vi "Add Library To Project.vi"(8 "error in":errorcluster, 11 "Msg Script Strategy in":refnum<class "Msg Script Strategy.lvclass">) -> (0 "error out":errorcluster)   [LabVIEW 2021, in "_Create From Template.lvlib" / "Script Strategy.lvlib" / "Msg Script Strategy.lvclass"]
uses:
  Msg Script Strategy.lvclass
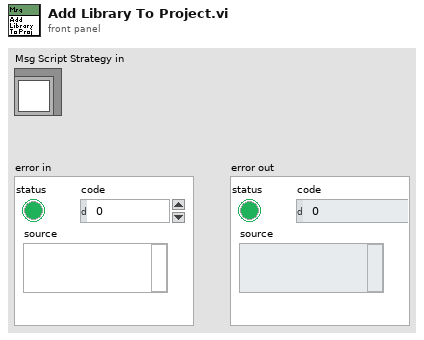
[diagram p1: front panel]
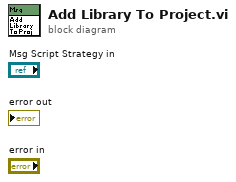
[diagram p0: block diagram]
diagram:
